vi "meas_dc_one_chanel.vi"(8 "error in (no error)":errorcluster, 10 "channel":u8(ring)=1 items=["1"=1, "2"=2, "3"=3, "4"=4, "5"=5, "6"=6, "7"=7, "8"=8, "9"=9, "10"=10, "11"=11, "12"=12, "13"=13, "14"=14, "15"=15, "16"=16, "17"=17, "18"=18, "19"=19, "20"=20], 11 "UI_out":T1) -> (0 "error out":errorcluster, 2 "Measurement":dbl, 3 "UI out":T1)   [LabVIEW 2017]
uses:
  ui.ctl
  classes/dc_power_supply/DC_power_supply.lvclass
  classes/report/Report.lvclass
  ui_buttons.ctl
  types/boc_type.ctl
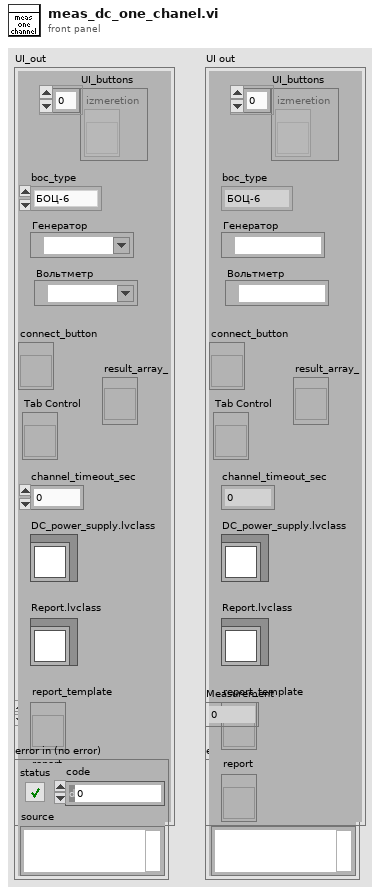
[diagram p1: front panel]
types:
  T1 = typedef "ui.ctl" = cluster{"UI_buttons":T2, "Tab Control":refnum<vi>, "connect_button":refnum<vi>, "generator":refnum<visa-resource-name>, "voltmetr":refnum<visa-resource-name>, "channel_timeout_sec":dbl, "boc_type":T3, "result_array_":refnum<vi>, "DC_power_supply.lvclass":refnum<class "DC_power_supply.lvclass">, "Report.lvclass":refnum<class "Report.lvclass">, "report_template":refnum<vi>, "report":refnum<vi>}
  T2 = typedef "ui_buttons.ctl" = refnum<vi>[]
  T3 = typedef "boc_type.ctl" = enum16{"БОЦ-6", "БОЦ-12"}
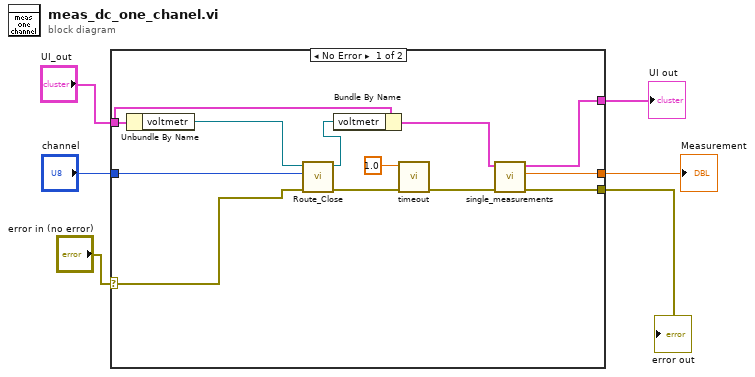
[diagram p0: block diagram]
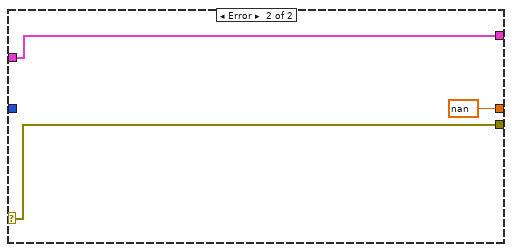
[diagram p2: hidden frame]
diagram:
  n1 = case shown="No Error" "error in (no error)" {
    selector: "error in (no error)" -> [w7 w20]
    tunnel: [w18 w20] -> w6
    tunnel: [w17 w21] -> w5
    tunnel: [w16 nan ("Measurement")] -> w4
    tunnel: "UI_out" -> [w12 w21]
    tunnel: "channel" -> [w8 _]
    frame No Error {
      n2 = Unbundle By Name(w12) -> ("voltmetr"=w9:refnum<visa-resource-name>)
      n3 = call <instrlib>:"Route_Close.vi"("error in (no error)"=w7, "channel"=w8, "VISA resource name"=w9) -> ("error out"=w10:errorcluster, "VISA resource name out"=w13:refnum<visa-resource-name>)  [unwired: 6 in, 1 out]
      n4 = Bundle By Name(cluster=w12, "voltmetr"=w13) -> (w14:T1)
      n5 = call "timeout.vi"("error in (no error)"=w10, "seconds to wait"=1.0) -> ("error IO"=w15:errorcluster)  [unwired: 9 in]
      n6 = call "single_measurements.vi"("error in (no error)"=w15, "UI in in"=w14) -> ("error out"=w18:errorcluster, "Measurement"=w16:dbl, "UI out"=w17:T1)  [unwired: 7 in]
    }
    frame Error {
    }
  }
  "error out" <- w6
  "UI out" <- w5
  "Measurement" <- w4
